vi "On Compile - Get Asynchronous Channels Status Block Refs.vi"(8 "error in":errorcluster, 11 "Item Ref":T1 format="%.0x") -> (0 "error out":errorcluster, 3 "Async Status Channels Refs":T2 {"VS Refs" format="%.0x"})   [LabVIEW 2020, in "Communication Bus Template System Explorer.lvlib" / "Implementation.lvlib"]
uses:
  Implementation.lvlib
  <vilib>/NI VeriStand/Custom Device API/Custom Device Item Ref.ctl
  <vilib>/NI VeriStand/Custom Device API/Custom Device API.lvlib
  <vilib>/NI VeriStand/Custom Device Tools/Custom Device Utility Library/Custom Device Utility Library.lvlib
  <vilib>/NI VeriStand/Custom Device Tools/Custom Device Utility Library/NI VeriStand - Search for Item by GUID.vi
  Scripting/Constants.vi
  Scripting/Communication Bus Template Scripting.lvlib
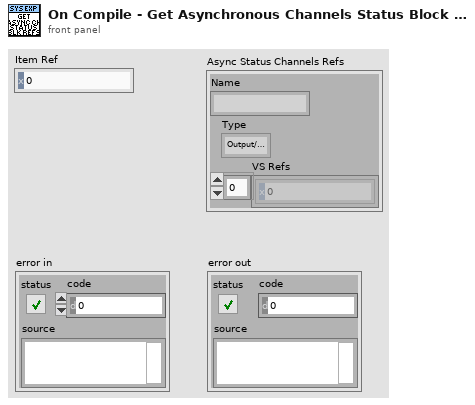
[diagram p1: front panel]
types:
  T1 = typedef "Custom Device API.lvlib/Custom Device Item Ref.ctl" = u64
  T2 = cluster{"Name":string, "Type":enum16{"Output/Write", "Input/Read", "Input/ReadWrite"}, "VS Refs":T1[]}
  T3 = enum16{"Output/Write", "Input/Read", "Input/ReadWrite"}
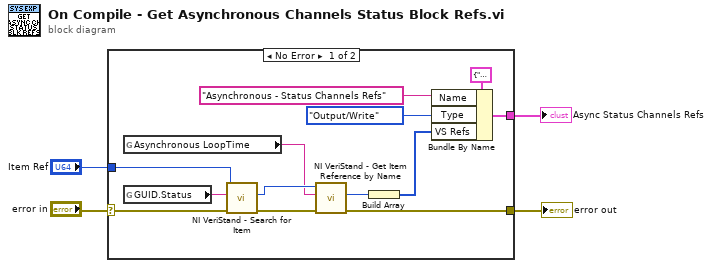
[diagram p0: block diagram]
diagram:
  n1 = case shown="No Error" "error in" {
    selector: "error in" -> [w9 w18]
    tunnel: "Item Ref" -> [w10 _]
    tunnel: [w11 w18] -> w2
    tunnel: [w14 _] -> w1
    frame No Error {
      n2 = global read "Constants.vi" "Asynchronous LoopTime"() -> (w5:string)
      n3 = global read "Constants.vi" "GUID.Status"() -> (w6:string)
      n4 = call-poly <vilib>:"NI VeriStand - Search for Item.vi"("error in"=w9, "Item GUID"=w6, "Section Ref in"=w10) -> ("error out"=w8:errorcluster, "Item Ref"=w7:T1)  [unwired: 5 in, 2 out]
      n5 = call <vilib>:"NI VeriStand - Get Item Reference by Name.vi"("error in (no error)"=w8, "Item Name"=w5, "Parent Ref in"=w7) -> ("error out"=w11:errorcluster, "Item Ref"=w17:T1)  [unwired: 5 in, 2 out]
      n6 = Build Array(w17) -> (w13:T1[])
      n7 = Bundle By Name(cluster=T2 {"Name"="", "Type"=enum."Output/Write", "VS Refs"=[]} ("Group"), "Name"="Asynchronous - Status Channels Refs", "Type"=T3."Output/Write", "VS Refs"=w13) -> (w14:T2)
    }
    frame Error {
    }
  }
  "error out" <- w2
  "Async Status Channels Refs" <- w1
